vi "FTW-Message-Lossy-Multipart-Initialize.vi"(0 "FTW-Message-Lossy In":refnum<class "FTW-Message-Lossy.lvclass">, 5 "Message":T1, 11 "error in":errorcluster) -> (4 "FTW-Message-Lossy Out":refnum<class "FTW-Message-Lossy.lvclass">, 6 "overflow?":bool, 15 "error out":errorcluster)   [LabVIEW 2015, in "FTW-Message-Lossy.lvclass"]
uses:
  FTW-Message-Lossy.lvclass
  Payload/FTW-MessagePayload.ctl
  FTW-Message-Lossy.lvclass/FTW-Message-Lossy.ctl
panel:
  # "Inputs"
  # "Outputs"
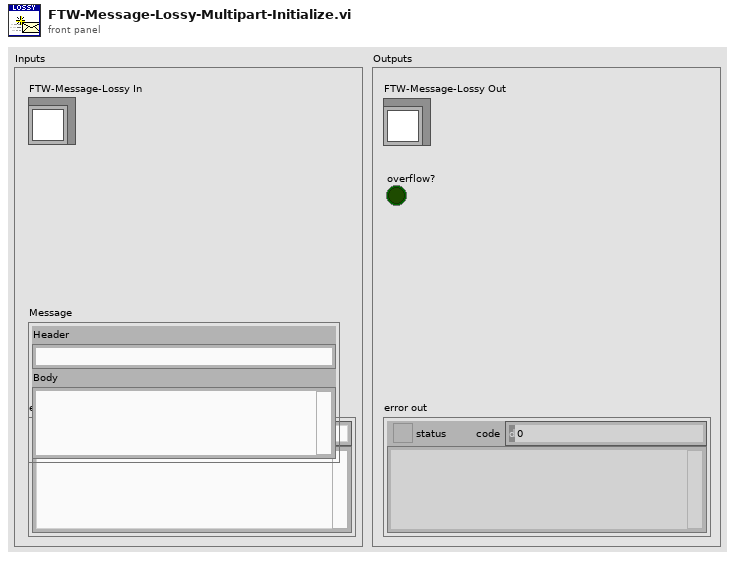
[diagram p1: front panel]
types:
  T1 = typedef "FTW-MessagePayload.ctl" = cluster{"Header":string, "Body":string, "FTW: Sender Identity":string, "FTW: Reply Address":string, "FTW: Reply Error":errorcluster}
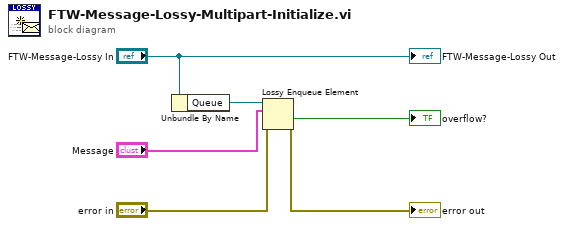
[diagram p0: block diagram]
diagram:
  n1 = Unbundle By Name("FTW-Message-Lossy In") -> ("Queue"=w1:refnum<queue>)
  n2 = Lossy Enqueue Element(queue=w1, element="Message", error in (no error)="error in") -> (overflow?=→"overflow?":bool, error out=→"error out":errorcluster)  [unwired: 2 out]
  "FTW-Message-Lossy Out" <- "FTW-Message-Lossy In"
